vi "Calc Inputs.vi"(8 "error in (no error)":errorcluster, 11 "Tare Calc in":refnum<class "Tare Calc.lvclass">) -> (0 "error out":errorcluster, 2 "Inputs":string[](array[string]))   [LabVIEW 2020, in "VolatusCalcs.lvlib" / "Tare Calc.lvclass"]
uses:
  Tare Calc.lvclass
  Tare Calc.lvclass/Tare Calc.ctl
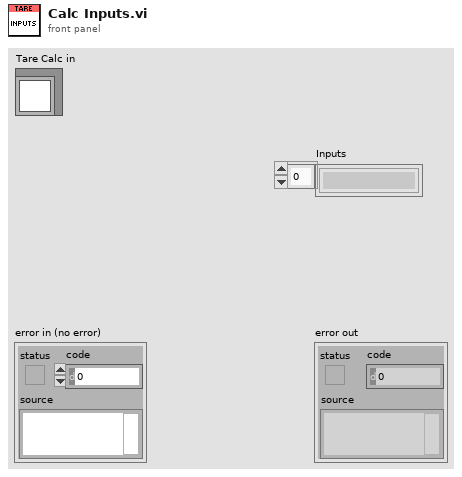
[diagram p1: front panel]
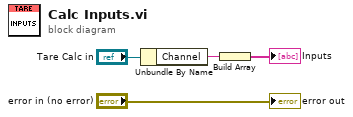
[diagram p0: block diagram]
diagram:
  n1 = Unbundle By Name("Tare Calc in") -> ("Channel"=w2:string)
  n2 = Build Array(w2) -> (→"Inputs":string[])
  "error out" <- "error in (no error)"
